vi "Map.vi"(7 "Action":enum8{"noop", "get", "set", "pop"}(ring), 10 "Queue in":refnum<queue>, 11 "Queue Name":string) -> (1 "Found?":bool, 2 "Queue out":refnum<queue>)   [LabVIEW 2018, in "Queue.lvlib"]
uses:
  Queue.lvlib
panel:
  # "Missing object. The object \"Map\" does not exist in the previous version."
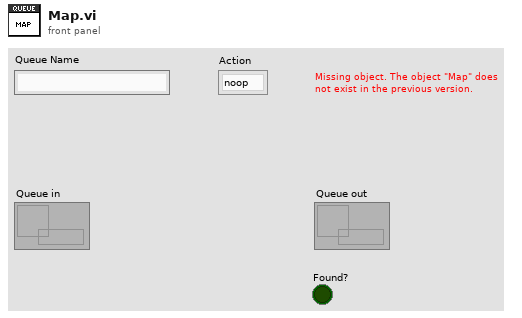
[diagram p1: front panel]
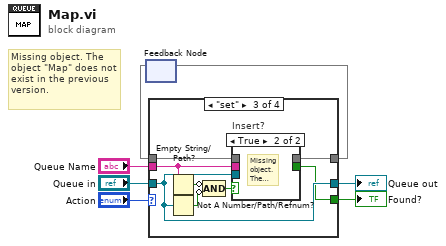
[diagram p0: block diagram]
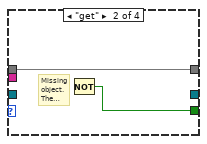
[diagram p3: hidden frame]
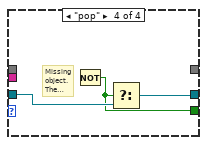
[diagram p5: hidden frame]
diagram:
  # "Missing object. The object \"Map\" does not exist in the previous version."
  n1 = feedback #1() -> (w5, w7)
  n2 = case shown="\"set\"" "Action" {
    tunnel: [w9 w12 w16 w24] -> w8
    tunnel: "Queue Name" -> [_ _ w21 w27]
    tunnel: w5 -> [w10 w13 w20 w29]
    tunnel: [w10 w13 w19 w28] -> w4
    tunnel: [_ w11 w14 w23] -> w3
    tunnel: "Queue in" -> [w9 _ w16 w26]
    frame "noop" {
    }
    frame "get" {
      # "Missing object. The object \"Look In Map\" does not exist in the previous version."
      n3 = Not() -> (.not. x?=w11:bool)  [unwired: 1 in]
    }
    frame "set" {
      n4 = Empty String/Path?(string/path=w21) -> (empty?=w18:bool)
      n5 = Not A Number/Path/Refnum?(number/path/refnum=w16) -> (NaN/Path/Refnum?=w15:bool)
      n6 = Compound Arithmetic op=AND(invert w18, invert w15) -> (w17:bool)
      n7 = case "Insert?" shown="True" w17 {
        tunnel: w20 -> [w22 _]
        tunnel: w16 -> [_ _]
        tunnel: w21 -> [_ _]
        tunnel: [w22 _] -> w19
        tunnel: [_ _] -> w14
        frame False {
        }
        frame True {
          # "Missing object. The object \"Insert Into Map\" does not exist in the previous version."
        }
      }
    }
    frame "pop" {
      # "Missing object. The object \"Remove From Map\" does not exist in the previous version."
      n8 = Not() -> (.not. x?=w23:bool)  [unwired: 1 in]
      n9 = Select(s=w23, f=w26) -> (t=w25:refnum<queue>, s? t:f=w24:refnum<queue>)
    }
  }
  "Queue out" <- w8
  "Found?" <- w3
  n10 = feedback-in #1(w4) -> ()
